vi "Get Data Set Size.vi"(8 "error in":errorcluster, 11 "Block Upload Initiate Transfer in":refnum<class "Block Upload Initiate Transfer.lvclass">) -> (0 "error out":errorcluster, 2 "Data Set Size":cluster{"Null":bool, "Value":u32}={"Null"=TRUE, "Value"=0}, 3 "Block Upload Initiate Transfer out":refnum<class "Block Upload Initiate Transfer.lvclass">)   [LabVIEW 2020, in "CANopen.lvlib" / "SDO Manager.lvlib" / "Block Upload Initiate Transfer.lvclass"]
uses:
  Block Upload Initiate Transfer.lvclass
  Block Upload Initiate Transfer.lvclass/Block Upload Initiate Transfer.ctl
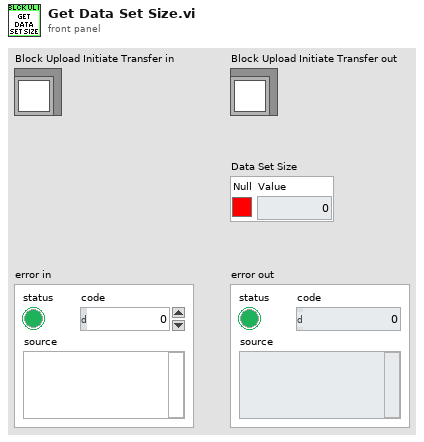
[diagram p1: front panel]
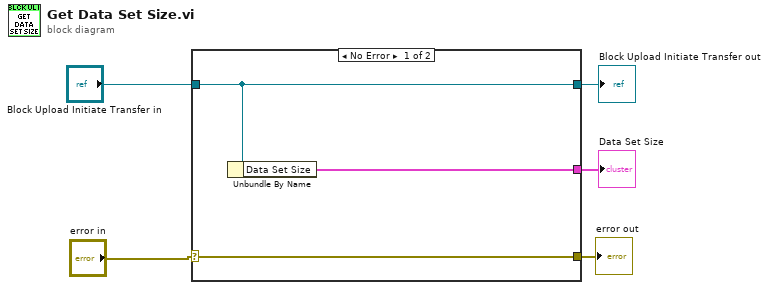
[diagram p0: block diagram]
diagram:
  n1 = case shown="No Error" "error in" {
    selector: "error in" -> [w8 w9]
    tunnel: [w8 w9] -> w2
    tunnel: [w7 w10] -> w4
    tunnel: "Block Upload Initiate Transfer in" -> [w7 w10]
    tunnel: [w6 _] -> w1
    frame No Error {
      n2 = Unbundle By Name(w7) -> ("Data Set Size"=w6:cluster{"Null":bool, "Value":u32})
    }
    frame Error {
    }
  }
  "error out" <- w2
  "Block Upload Initiate Transfer out" <- w4
  "Data Set Size" <- w1
